vi "init_img_processing_vars.vi"(0 "Region of interest":i32[](array[numeric]), 7 "Count Buffer Size":i32=2000000) -> (4 "Image Data Out":T1, 8 "Count Total Q Out":T2)   [LabVIEW 2023]
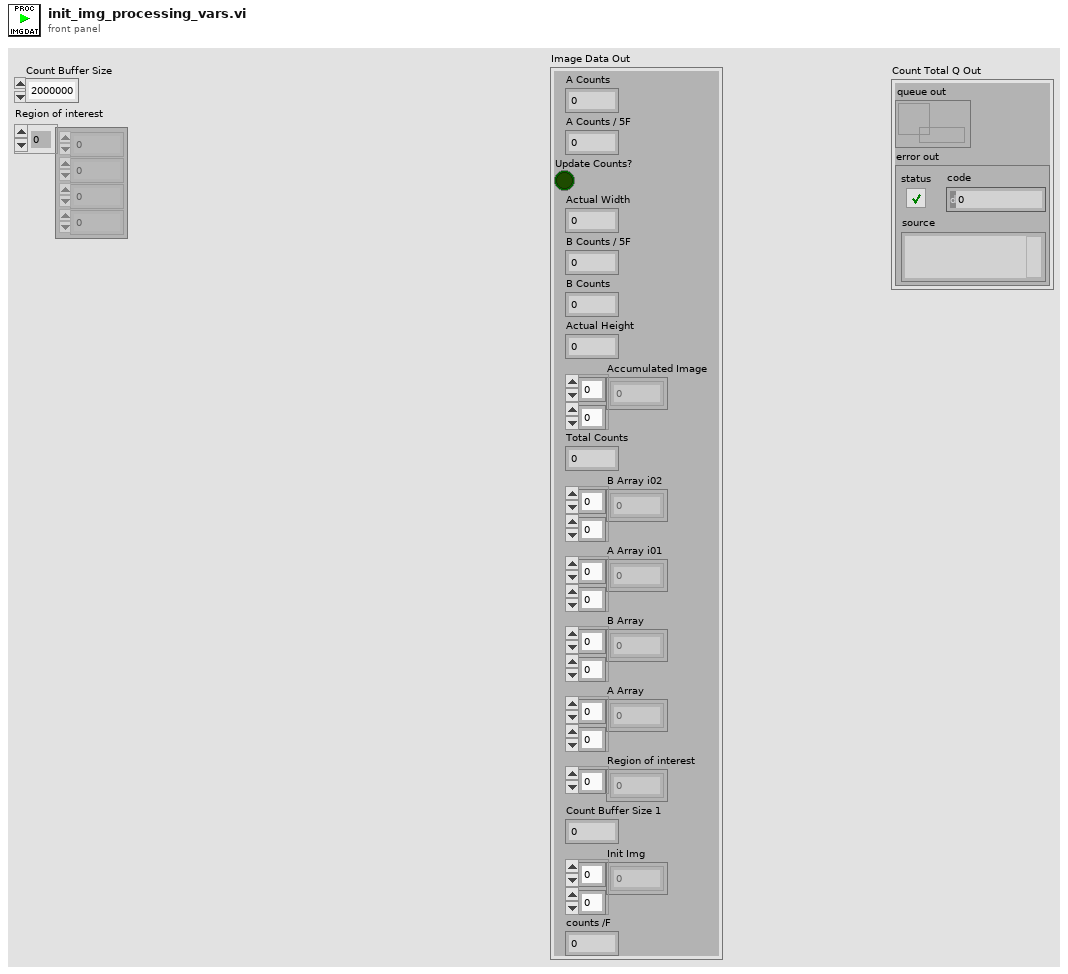
[diagram p1: front panel]
types:
  T1 = cluster{"A Counts":i32, "A Counts / 5F":dbl, "Update Counts?":bool, "Actual Width":u32, "B Counts / 5F ":dbl, "B Counts":i32, "Actual Height":u32, "Accumulated Image ":i16[][], "Total Counts":i32, "B Array i02":sgl[][], "A Array i01":sgl[][], "B Array":i16[][], "A Array":i16[][], "Region of interest":i32[], "Count Buffer Size 1":i32, "Init Img":i16[][], "counts /F":i16}
  T2 = cluster{"queue out":refnum<queue>, "error out":errorcluster}
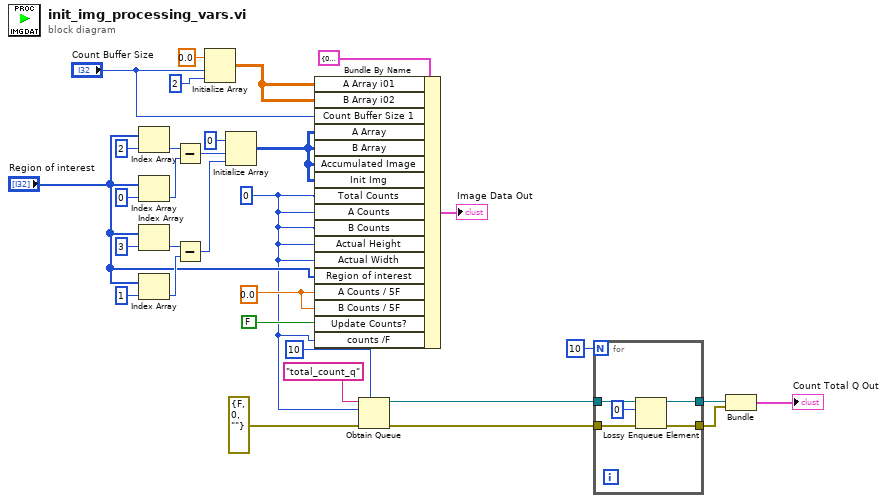
[diagram p0: block diagram]
diagram:
  w10 = 0.0 ("A Counts / 5F")
  w8 = 0 ("Total Counts")
  n1 = Index Array(array="Region of interest", index=2) -> (element=w26:i32)
  n2 = Index Array(array="Region of interest", index=0) -> (element=w25:i32)
  n3 = Index Array(array="Region of interest", index=3) -> (element=w24:i32)
  n4 = Index Array(array="Region of interest", index=1) -> (element=w23:i32)
  n5 = Subtract(x=w26, y=w25) -> (x-y=w21:i32)
  n6 = Subtract(x=w24, y=w23) -> (x-y=w20:i32)
  n7 = Initialize Array(sgl 0.0 ("element"), "Count Buffer Size", 2 ("dimension size")) -> (w17:sgl[][])
  n8 = Initialize Array(i16 0 ("element"), w21, w20) -> (w12:i16[][])
  n9 = Bundle By Name(cluster=T1 {"A Counts"=0, "A Counts / 5F"=0.0, "Update Counts?"=FALSE, "Actual Width"=0, "B Counts / 5F "=0.0, "B Counts"=0, "Actual Height"=0, "Accumulated Image "=[], "Total Counts"=0, "B Array i02"=[], "A Array i01"=[], "B Array"=[], "A Array"=[], "Region of interest"=[0, 0, 1020, 1020], "Count Buffer Size 1"=2000000, "Init Img"=[], "counts /F"=0}, "A Array i01"=w17, "B Array i02"=w17, "Count Buffer Size 1"="Count Buffer Size", "A Array"=w12, "B Array"=w12, "Accumulated Image"=w12, "Init Img"=w12, "Total Counts"=w8, "A Counts"=w8, "B Counts"=w8, "Actual Height"=w8, "Actual Width"=w8, "Region of interest"="Region of interest", "A Counts / 5F"=w10, "B Counts / 5F"=w10, "Update Counts?"=FALSE, "counts /F"=w8) -> (→"Image Data Out":T1)
  n10 = Obtain Queue(max queue size (-1, unlimited)=10, name (unnamed)="total_count_q", element data type=w8, error in (no error)=errorcluster {"status"=FALSE, "code"=0, "source"=""}) -> (queue out=w6:refnum<queue>, error out=w5:errorcluster)  [unwired: 1 in, 1 out]
  n11 = for {
    N: 10 -> [_]
    tunnel: w6 -> [w36]
    tunnel: w5 -> [w35]
    tunnel: [w33] -> w4
    tunnel: [w34] -> w3
    n12 = Lossy Enqueue Element(queue=w36, element=0, error in (no error)=w35) -> (queue out=w33:refnum<queue>, error out=w34:errorcluster)  [unwired: 2 out]
  }
  n13 = Bundle("queue out"=w4, "error out"=w3) -> (→"Count Total Q Out":T2)  [unwired: 1 in]
